vi "Minimax.vi"(0 "Game":i32[][](array[numeric]), 1 "Active Turn":i32=1, 2 "Depth":i32, 5 "NextTurn":i32=1) -> (14 "Score":i32, 15 "Next Move":cluster{"Row":i32, "Col":i32}, 17 "Scores":i32[](array[numeric]), 18 "Moves":cluster{"Row":i32, "Col":i32}[](array[cluster]))   [LabVIEW 2017]
panel:
  in  "Max Depth (7)":i32=7 min=7 max=23
  # "3x3 Felder Max Depth 7\n4*4 Felder Max Depth 15\n5*5 Felder Max Depth 23"
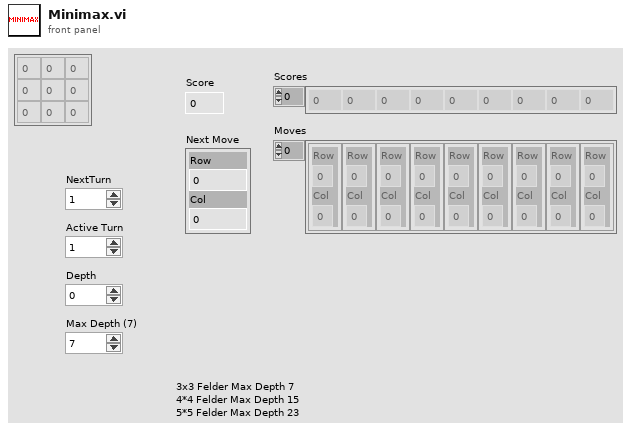
[diagram p1: front panel]
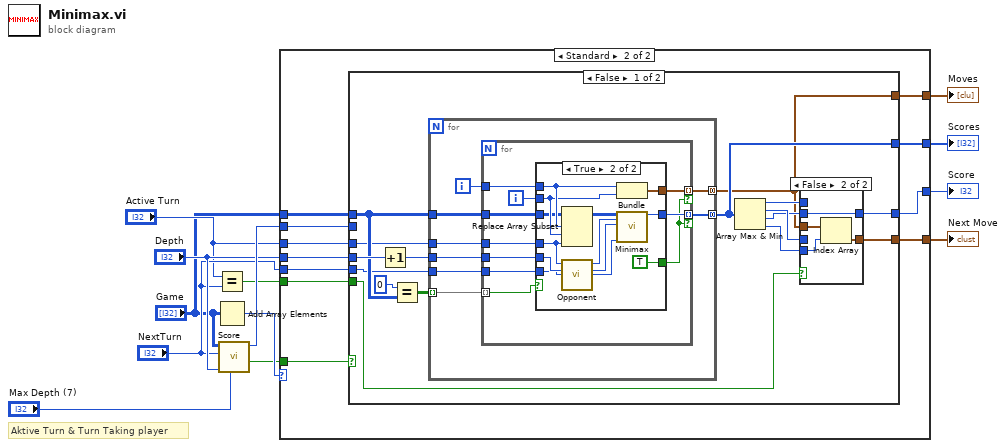
[diagram p0: block diagram]
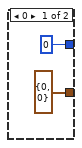
[diagram p2: hidden frame]
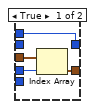
[diagram p3: hidden frame]
diagram:
  # "Aktive Turn & Turn Taking player"
  n1 = Equal?(x="Active Turn", y="NextTurn") -> (x = y?=w8:bool)
  n2 = Add Array Elements(numeric array="Game") -> (sum=w3:i32)
  n3 = call "Score.vi"("Max Depth (8)"="Max Depth (7)", "Depth"="Depth", "Turn Taking Player"="NextTurn", "Game"="Game") -> ("Game over"=w1:bool, "Score"=w12:i32)  [unwired: 5 in, 1 out]
  n4 = case shown="Standard" w3 {
    tunnel: [0 ("Score") w26] -> w13
    tunnel: w12 -> [_ w25]
    tunnel: [cluster{"Row":i32, "Col":i32} {"Row"=0, "Col"=0} ("Move") w24] -> w11
    tunnel: [_ w23] -> w10
    tunnel: [_ w22] -> w9
    tunnel: w8 -> [_ w21]
    tunnel: "Depth" -> [_ w20]
    tunnel: "NextTurn" -> [_ w19]
    tunnel: "Active Turn" -> [_ w18]
    tunnel: w1 -> [_ w17]
    tunnel: "Game" -> [_ w16]
    frame 0 {
    }
    frame Default {
      n5 = case shown="False" w17 {
        tunnel: [w33 w80] -> w26
        tunnel: w25 -> [_ w80]
        tunnel: w20 -> [w42 _]
        tunnel: w16 -> [w39 _]
        tunnel: w18 -> [w37 _]
        tunnel: [w34 _] -> w24
        tunnel: [w30 _] -> w22
        tunnel: [w29 _] -> w23
        tunnel: w19 -> [w28 _]
        tunnel: w21 -> [w27 _]
        frame False {
          n6 = Increment(x=w42) -> (x+1=w38:i32)
          n7 = Equal?(x=0, y=w39) -> (x = y?=w40:bool[][])
          n8 = for {
            tunnel: w40 -> [w58] mode=indexing
            tunnel: w39 -> [w56]
            tunnel: w38 -> [w55]
            tunnel: w37 -> [w52]
            tunnel: w28 -> [w51]
            tunnel: [w54] -> w30 mode=concatenating
            tunnel: [w53] -> w29 mode=concatenating
            i -> [w57]
            n9 = for {
              tunnel: w58 -> [w68] mode=indexing
              tunnel: w57 -> [w66]
              tunnel: w56 -> [w67]
              tunnel: w55 -> [w64]
              tunnel: w52 -> [w61]
              tunnel: w51 -> [w60]
              tunnel: [w63] -> w54 mode=indexing if=w59
              tunnel: [w62] -> w53 mode=indexing if=w59
              i -> [w65]
              n10 = case shown="True" w68 {
                tunnel: w67 -> [_ w70]
                tunnel: w66 -> [_ w78]
                tunnel: w65 -> [_ w77]
                tunnel: w64 -> [_ w79]
                tunnel: [_ w73] -> w63
                tunnel: [_ w72] -> w62
                tunnel: w61 -> [_ w75]
                tunnel: w60 -> [_ w76]
                tunnel: [_ TRUE] -> w59
                frame False {
                }
                frame True {
                  n11 = Replace Array Subset(array=w70, new element=w75, index (row)=w78, index (col)=w77) -> (w69:i32[][])
                  n12 = call "Opponent.vi"("Player"=w75) -> ("Opponent"=w74:i32)  [unwired: 10 in]
                  n13 = Bundle(w78, w77) -> (w72:cluster{i32, i32})  [unwired: 1 in]
                  n14 = call "Minimax.vi"("Game"=w69, "Active Turn"=w74, "Depth"=w79, "NextTurn"=w76) -> ("Score"=w73:i32)  [unwired: 12 in, 3 out]
                }
              }
            }
          }
          n15 = Array Max & Min(array=w30) -> (max value=w32:i32, max index (indices)=w36:i32, min value=w31:i32, min index (indices)=w35:i32)
          n16 = case shown="False" w27 {
            tunnel: w29 -> [w46 w50]
            tunnel: w36 -> [w43 _]
            tunnel: w35 -> [_ w47]
            tunnel: [w45 w49] -> w34
            tunnel: [w44 w48] -> w33
            tunnel: w32 -> [w44 _]
            tunnel: w31 -> [_ w48]
            frame True {
              n17 = Index Array(array=w46, index=w43) -> (element=w45:cluster{i32, i32})
            }
            frame False {
              n18 = Index Array(array=w50, index=w47) -> (element=w49:cluster{i32, i32})
            }
          }
        }
        frame True {
        }
      }
    }
  }
  "Score" <- w13
  "Next Move" <- w11
  "Scores" <- w9
  "Moves" <- w10
